vi "RFH-View-simple.vi"() -> ()   [LabVIEW 2020, in "RFH-Reflection_File_Handler.lvlib"]
uses:
  RFH-Reflection_File_Handler.lvlib
panel:
  out "Reflection Imag":T1(graph)
  in  "Folder Path":path
  out "Reflection Real":T1(graph)
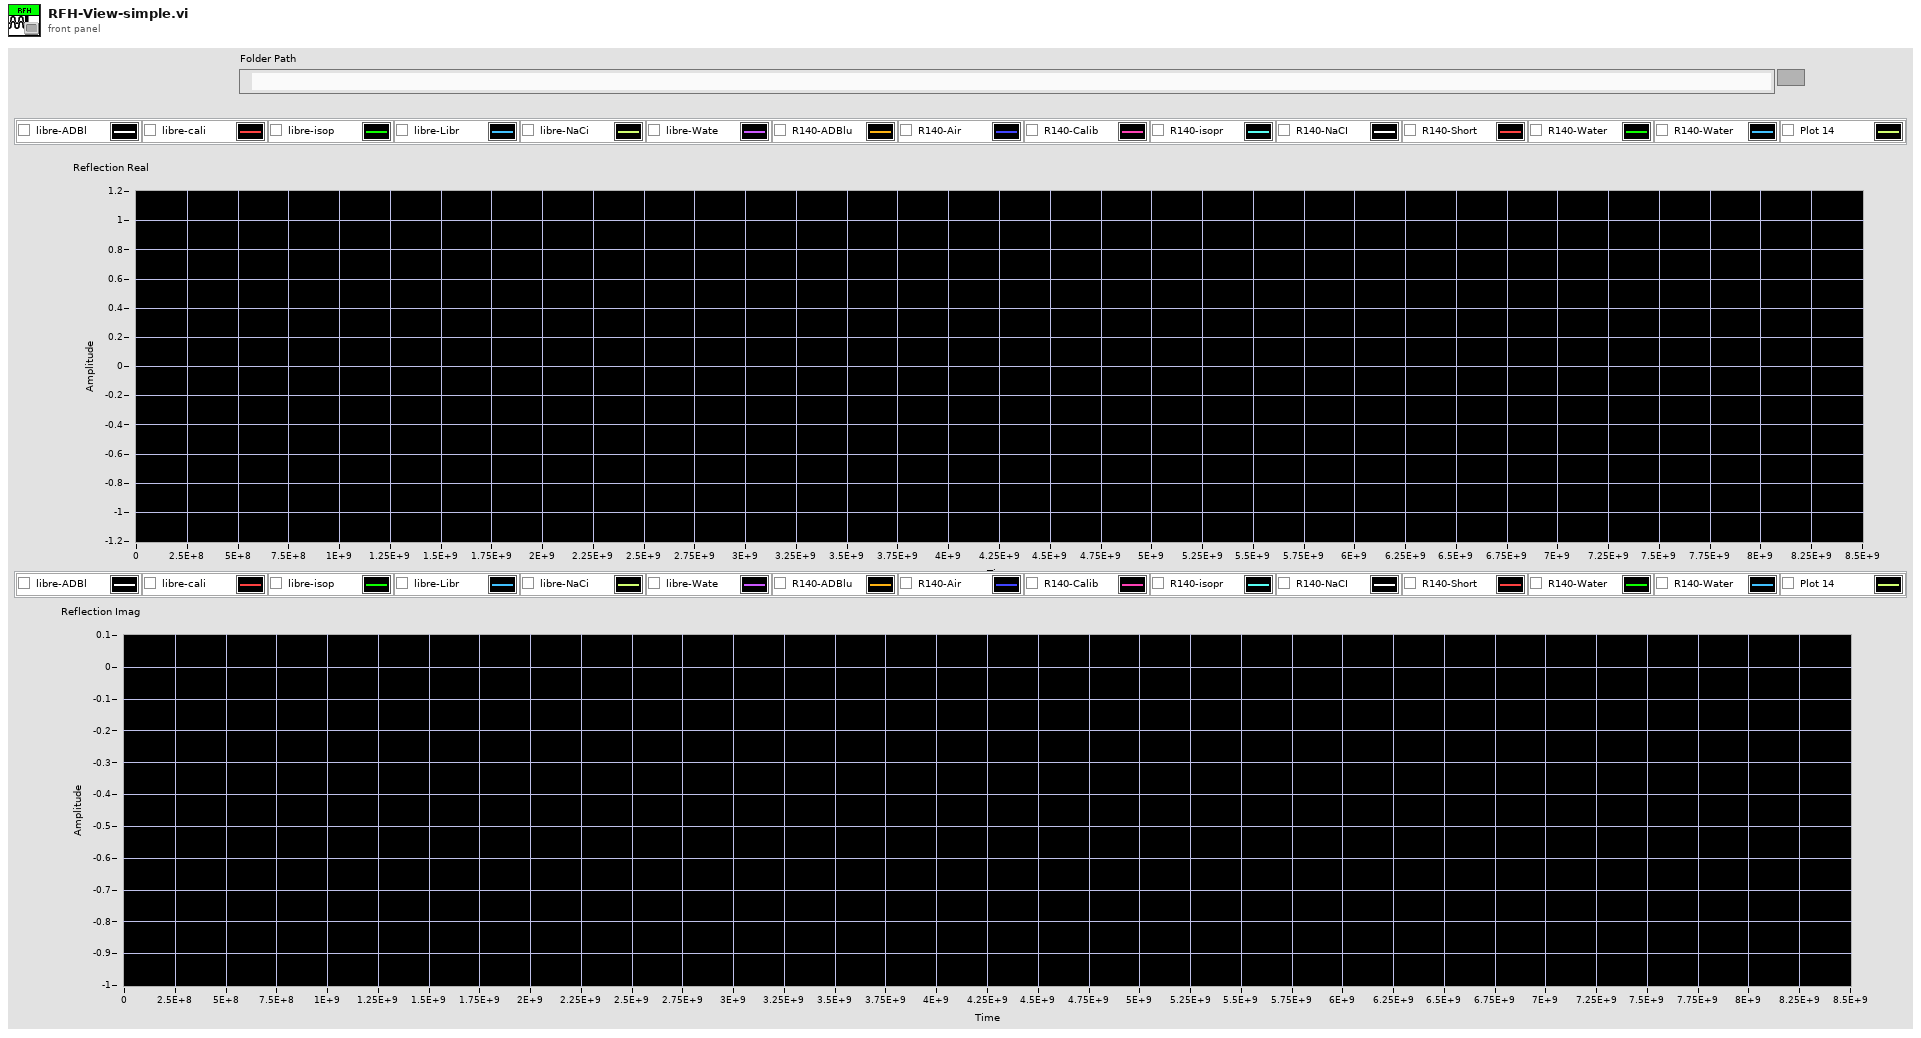
[diagram p1: front panel]
types:
  T1 = cluster{"Frequency":dbl[], "Reflection'":dbl[]}[]
  T2 = typedef "RFH-Reflection_File_Handler.lvlib/RFH-common_data_format.ctl" = cluster{"Frequency":dbl[], "Reflection'":dbl[], "Reflection''":dbl[], "Permativity'":dbl[], "Permativity''":dbl[]}
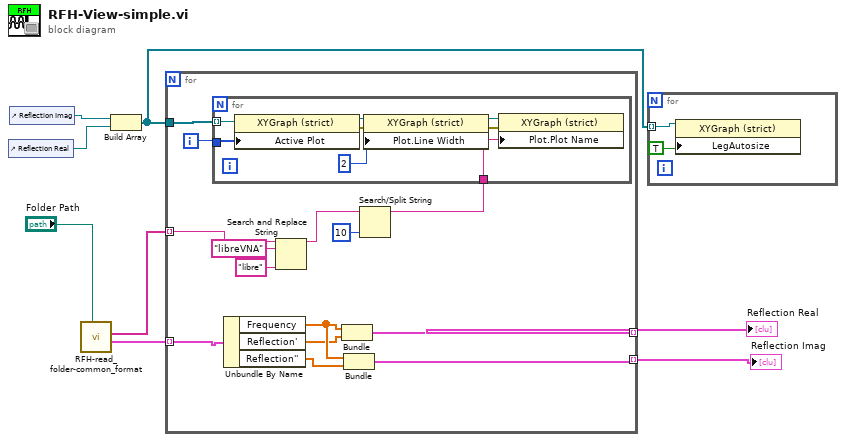
[diagram p0: block diagram]
diagram:
  n1 = control-ref of="Reflection Real"() -> (w2:refnum<vi>)
  n2 = control-ref of="Reflection Imag"() -> (w3:refnum<vi>)
  n3 = call "RFH-read_folder-common_format.vi"("Folder Path"="Folder Path") -> ("Data"=w8:T2[], "Names"=w5:string[])  [unwired: 9 in]
  n4 = Build Array(w3, w2) -> (w1:refnum<vi>[])
  n5 = for {
    tunnel: w8 -> [w22] mode=indexing
    tunnel: [w18] -> w7 mode=indexing
    tunnel: [w17] -> w4 mode=indexing
    tunnel: w5 -> [w13] mode=indexing
    tunnel: w1 -> [w9]
    i -> [w16]
    n6 = Unbundle By Name(w22) -> ("Frequency"=w21:dbl[], "Reflection'"=w20:dbl[], "Reflection''"=w19:dbl[])
    n7 = Search and Replace String(input string=w13, search string="libreVNA", replace string="libre" ("replace string (\"\")")) -> (result string=w10:string)  [unwired: 5 in, 3 out]
    n8 = Bundle("Frequency"=w21, "Reflection'"=w20) -> (w18:cluster{"Frequency":dbl[], "Reflection'":dbl[]})  [unwired: 1 in]
    n9 = Bundle("Frequency"=w21, "Reflection''"=w19) -> (w17:cluster{"Frequency":dbl[], "Reflection''":dbl[]})  [unwired: 1 in]
    n10 = Search/Split String(string=w10, offset (0)=10) -> (substring before match=w14:string)  [unwired: 1 in, 2 out]
    n11 = for {
      tunnel: w16 -> [w29]
      tunnel: w14 -> [w26]
      tunnel: w9 -> [w25] mode=indexing
      n12 = property on="Property Node" class="XYGraph (strict)"(reference=w25, "Active Plot"=w29) -> (reference out=w24:refnum<vi>, error out=w30:errorcluster)  [unwired: 1 in]
      n13 = property on="Property Node" class="XYGraph (strict)"(reference=w24, error in=w30, "Plot.Line Width"=u8 2) -> (reference out=w23:refnum<vi>, error out=w28:errorcluster)
      n14 = property on="Property Node" class="XYGraph (strict)"(reference=w23, error in=w28, "Plot.Plot Name"=w26) -> ()  [unwired: 2 out]
    }
  }
  "Reflection Real" <- w7
  "Reflection Imag" <- w4
  n15 = for {
    tunnel: w1 -> [w31] mode=indexing
    n16 = property on="Property Node" class="XYGraph (strict)"(reference=w31, "LegAutosize"=TRUE ("Legend:Autosize")) -> ()  [unwired: 1 in, 2 out]
  }
